vi "Plot histogram.vi"() -> ()   [LabVIEW 2010]
uses:
  <vilib>/Analysis/NI_AALBase.lvlib
panel:
  in  "Results file Out":path
  in  "intervals":i32=1
  out "Waveform Graph":i32[](graph)
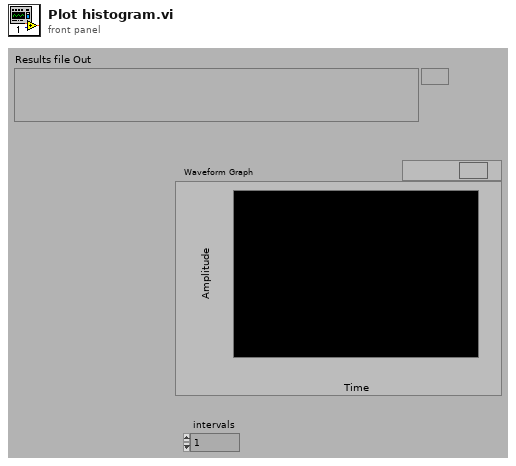
[diagram p1: front panel]
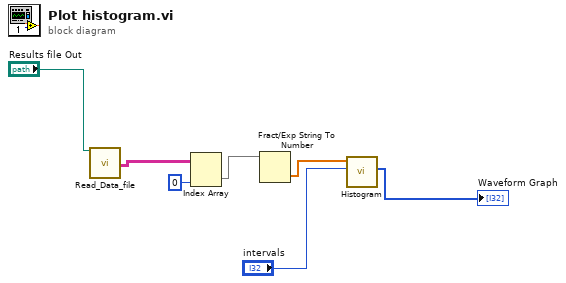
[diagram p0: block diagram]
diagram:
  n1 = call "Read_Data_file.vi"("Results file"="Results file Out") -> ("Channel Values Out"=w7:string[][])  [unwired: 9 in, 9 out]
  n2 = Index Array(array=w7, index (col)=0 ("disabled index (col)")) -> (element=w5:string[])  [unwired: 1 in]
  n3 = Fract/Exp String To Number(string=w5) -> (number=w4:dbl[])  [unwired: 3 in, 1 out]
  n4 = call <vilib>:"Histogram.vi"("intervals"="intervals", "X"=w4) -> ("Histogram: h(x)"=→"Waveform Graph":i32[])  [unwired: 6 in, 3 out]
